vi "Header String.vi"(8 "error in (no error)":errorcluster, 11 "Response in":refnum<class "Response.lvclass">) -> (0 "error out":errorcluster, 2 "Header String":string, 3 "Response out":refnum<class "Response.lvclass">)   [LabVIEW 2020, in "HTTP Utils.lvlib" / "Response.lvclass"]
uses:
  Response.lvclass
  Response.lvclass/Response.ctl
  Cookie/Cookie.lvclass
  HTTP Utils.lvlib
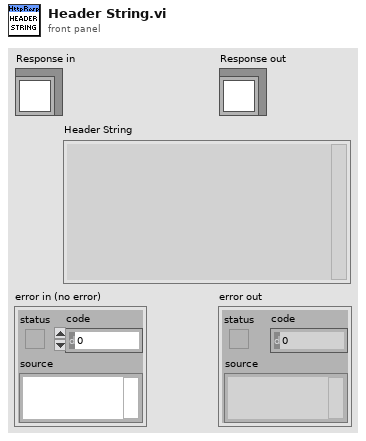
[diagram p1: front panel]
types:
  T1 = typedef "HTTP Utils.lvlib/Cookie Map.ctl" = map{string, refnum<class "Cookie.lvclass">}
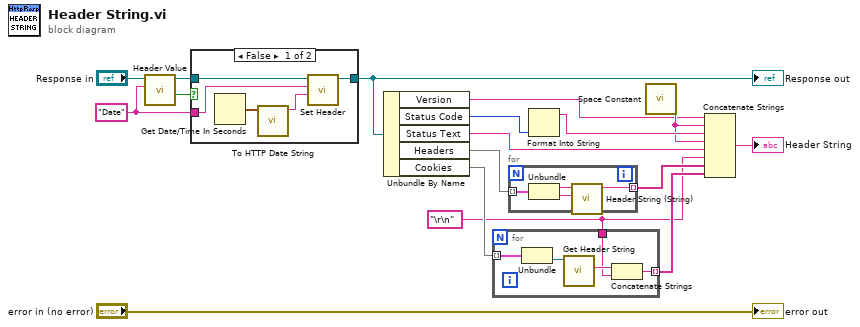
[diagram p0: block diagram]
diagram:
  w1 = "Date" ("Header")
  w7 = "\r\n" ("string")
  n1 = call "Header Value.vi"("Header"=w1, "Response in"="Response in") -> ("Exists"=w4:bool, "Response out"=w3:refnum<class "Response.lvclass">)  [unwired: 6 in, 2 out]
  n2 = case shown="False" w4 {
    tunnel: w3 -> [w22 w23]
    tunnel: [w21 w23] -> w2
    tunnel: w1 -> [w20 _]
    frame False {
      n3 = Get Date/Time In Seconds() -> (seconds since 1Jan1904=w19:timestamp)
      n4 = call "To HTTP Date String.vi"("Time Stamp"=w19) -> ("HTTP Date"=w18:string)  [unwired: 10 in]
      n5 = call "Set Header.vi"("Value"=w18, "Header"=w20, "Response in"=w22) -> ("Response out"=w21:refnum<class "Response.lvclass">)  [unwired: 6 in, 2 out]
    }
    frame True {
    }
  }
  "Response out" <- w2
  n6 = Unbundle By Name(w2) -> ("Version"=w10:string, "Status Code"=w13:u16, "Status Text"=w14:string, "Headers"=w16:map{string, string}, "Cookies"=w9:T1)
  n7 = for {
    tunnel: w9 -> [w28] mode=indexing
    tunnel: [w27] -> w8 mode=indexing
    tunnel: w7 -> [w24]
    n8 = Unbundle(w28) -> ("Cookie"=w26:refnum<class "Cookie.lvclass">)  [unwired: 1 out]
    n9 = call "Get Header String.vi"("Cookie in"=w26) -> ("Header String"=w25:string)  [unwired: 8 in, 2 out]
    n10 = Concatenate Strings(w25, w24) -> (w27:string)
  }
  n11 = for {
    tunnel: w16 -> [w32] mode=indexing
    tunnel: [w29] -> w15 mode=indexing
    n12 = Unbundle(w32) -> (w31:string, w30:string)
    n13 = call "Header String (String).vi"("Value"=w30, "Name"=w31) -> ("Header"=w29:string)  [unwired: 9 in]
  }
  n14 = Format Into String(w13) -> (resulting string=w12:string)  [unwired: 3 in, 1 out]
  n15 = call <vilib>:"Space Constant.vi"() -> ("String"=w11:string)
  n16 = Concatenate Strings(w10, w11, w12, w11, w14, w7, w15, w8) -> (→"Header String":string)
  "error out" <- "error in (no error)"
